vi "JKISM++ Destroy Global Log Event.vi"(8 "Error in":errorcluster caption="Error in (no error)", 11 "JKISM Global Log Event":refnum<user-event>) -> (0 "Error out":errorcluster)   [LabVIEW 2014, in "JKI-State-Machine-Plus.lvlib"]
uses:
  JKI-State-Machine-Plus.lvlib
  _Support/Typedef/_JKI StateMachine Current State.ctl
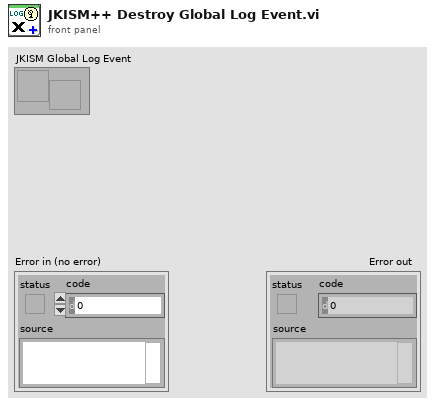
[diagram p1: front panel]
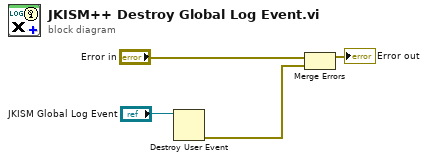
[diagram p0: block diagram]
diagram:
  n1 = Destroy User Event(user event="JKISM Global Log Event") -> (error out=w4:errorcluster)  [unwired: 1 in]
  n2 = Merge Errors("Error in", w4) -> (→"Error out":errorcluster)
